vi "check slipping wheels.vi"(10 "Matriz m \nesperada":T1, 11 "Matriz m\nobservada":T1) -> (1 "m sem\ndeslizamento":T1, 3 "m sem \ndeslizamento \ne no \nsentido \noriginal":dbl[](array[numeric]), 5 "deslizamento?":bool)   [LabVIEW 2016]
uses:
  <vilib>/Analysis/Matrix/Datatypes/RealMatrix.ctl
  <vilib>/Analysis/Matrix/Numeric/Multiply/Multiply - RM,RM.vi
  <vilib>/Analysis/Matrix/Numeric/Conversions/Matrix To Array - RM.vi
  <vilib>/Analysis/Matrix/NI_Matrix.lvlib
panel:
  out "Produto":dbl
  out "(I-B*D) * m":T1
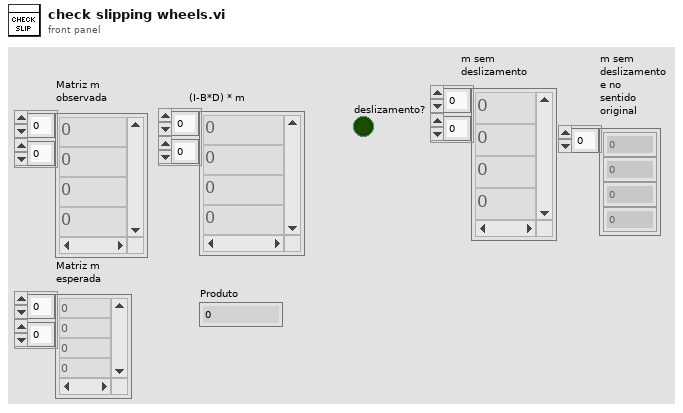
[diagram p1: front panel]
types:
  T1 = typedef "NI_Matrix.lvlib/RealMatrix.ctl" = dbl[][]
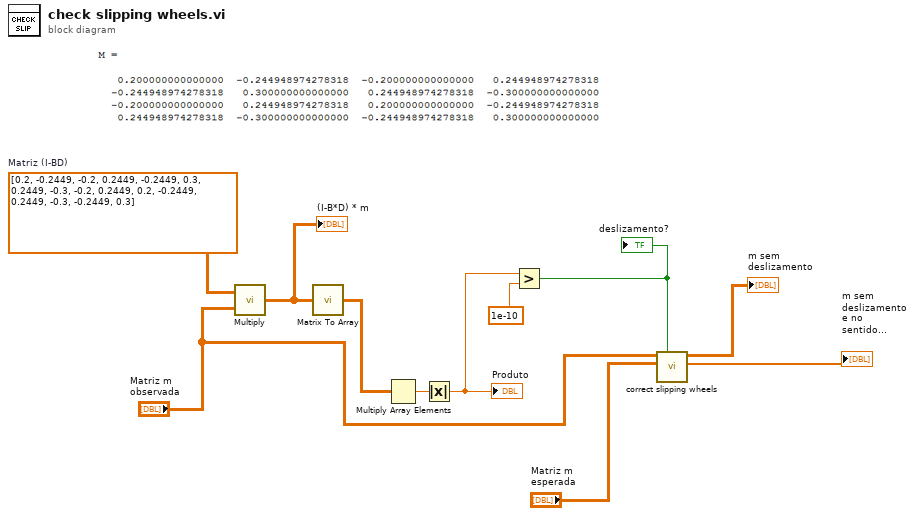
[diagram p0: block diagram]
diagram:
  w11 = T1 [[0.2, -0.2449, -0.2, 0.2449], [-0.2449, 0.3, 0.2449, -0.3], [-0.2, 0.2449, 0.2, -0.2449], [0.2449, -0.3, -0.2449, 0.3]]  # Matriz (I-BD)
  n1 = call-poly <vilib>:"Multiply.vi"("Real Matrix B"="Matriz m\nobservada", "Real Matrix A"=w11) -> ("A * B"=w10:T1)
  "(I-B*D) * m" <- w10
  n2 = call-poly <vilib>:"Matrix To Array.vi"("Real Matrix"=w10) -> ("Real 2D Array"=w9:dbl[][])
  n3 = Multiply Array Elements(1:w9) -> (0:w7:dbl)
  n4 = Absolute Value(x=w7) -> (abs(x)=w6:dbl)
  "Produto" <- w6
  n5 = Greater?(x=w6, y=1e-10) -> (0:w5:bool)
  "deslizamento?" <- w5
  n6 = call "correct slipping wheels.vi"("deslizamento?"=w5, "Matriz m \nesperada"="Matriz m \nesperada", "Matriz m\nobservada"="Matriz m\nobservada") -> ("m sem \ndeslizamento \ne no \nsentido \noriginal"=→"m sem \ndeslizamento \ne no \nsentido \noriginal":dbl[], "m sem\ndeslizamento"=→"m sem\ndeslizamento":T1)  [unwired: 7 in]
